vi "校准任务设置.vi"(10 "校准触发任务":refnum<user-event>, 11 "用户事件":refnum<user-event>) -> ()   [LabVIEW 2016, in "斯坦道CODMn新电路板.lvlib"]
uses:
  <vilib>/Utility/xml.llb/Write to XML File(string).vi
  <vilib>/Utility/xml.llb/Read From XML File(string).vi
panel:
  in  "导入":bool
  in  "保存":bool
  in  "校准任务存档":T1[](array[typedef])
  out "字符串":string
  out "校准运行状态":bool
  in  "校准任务":T1[](array[typedef])
  in  "停止":bool
  in  "设置":bool
  in  "执行":bool
  in  "删除":bool
  in  "清空":bool
  in  "任务列表":i32(listbox)
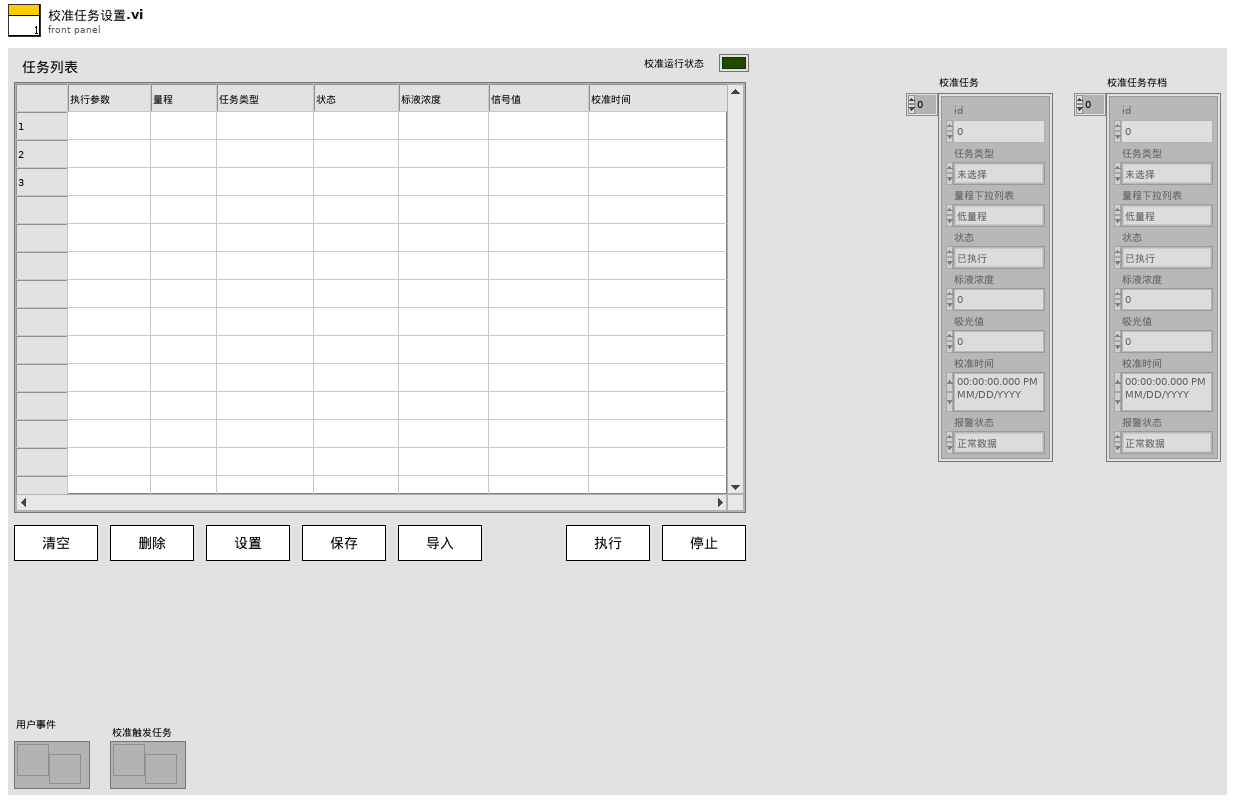
[diagram p1: front panel]
types:
  T1 = typedef "校准任务.ctl" = cluster{"id":u16, "任务类型":enum16{"未选择", "空白校准", "标样校准", "标样核查", "零点核查", "跨度核查"}, "量程下拉列表":enum16{"低量程", "高量程"}, "状态":enum16{"已执行", "待执行", "执行中", "停止"}, "标液浓度":dbl, "吸光值":dbl, "校准时间":timestamp, "报警状态":enum16{"正常数据", "报警数据"}}
  T2 = cluster{"校准类型":string, "校准数据":cluster{"时间":timestamp, "标液值":dbl, "检测值":dbl, "吸光值":dbl}}
  T3 = enum8{"Enabled", "Disabled", "Disabled and Grayed Out"}
  T4 = typedef "LVPoint32TypeDef.ctl" = cluster{"Horizontal":i32, "Vertical":i32}
  T5 = typedef "LVRowAndColumnTypeDef.ctl" = cluster{"Row":i32, "Column":i32}
  T6 = enum16{"未选择", "空白校准", "标样校准", "标样核查", "零点核查", "跨度核查"}
  T7 = cluster{"id":u16, "任务类型":enum16{"未选择", "空白校准", "标样校准", "标样核查", "零点核查", "跨度核查"}, "量程下拉列表":enum16{"低量程", "高量程"}, "状态":enum16{"已执行", "待执行", "执行中", "停止"}, "标液浓度":dbl, "吸光值":dbl, "校准时间":timestamp, "报警状态":enum16{"正常数据", "报警数据"}}
  T8 = enum32{"Bad", "Idle", "Run top level", "Running"}
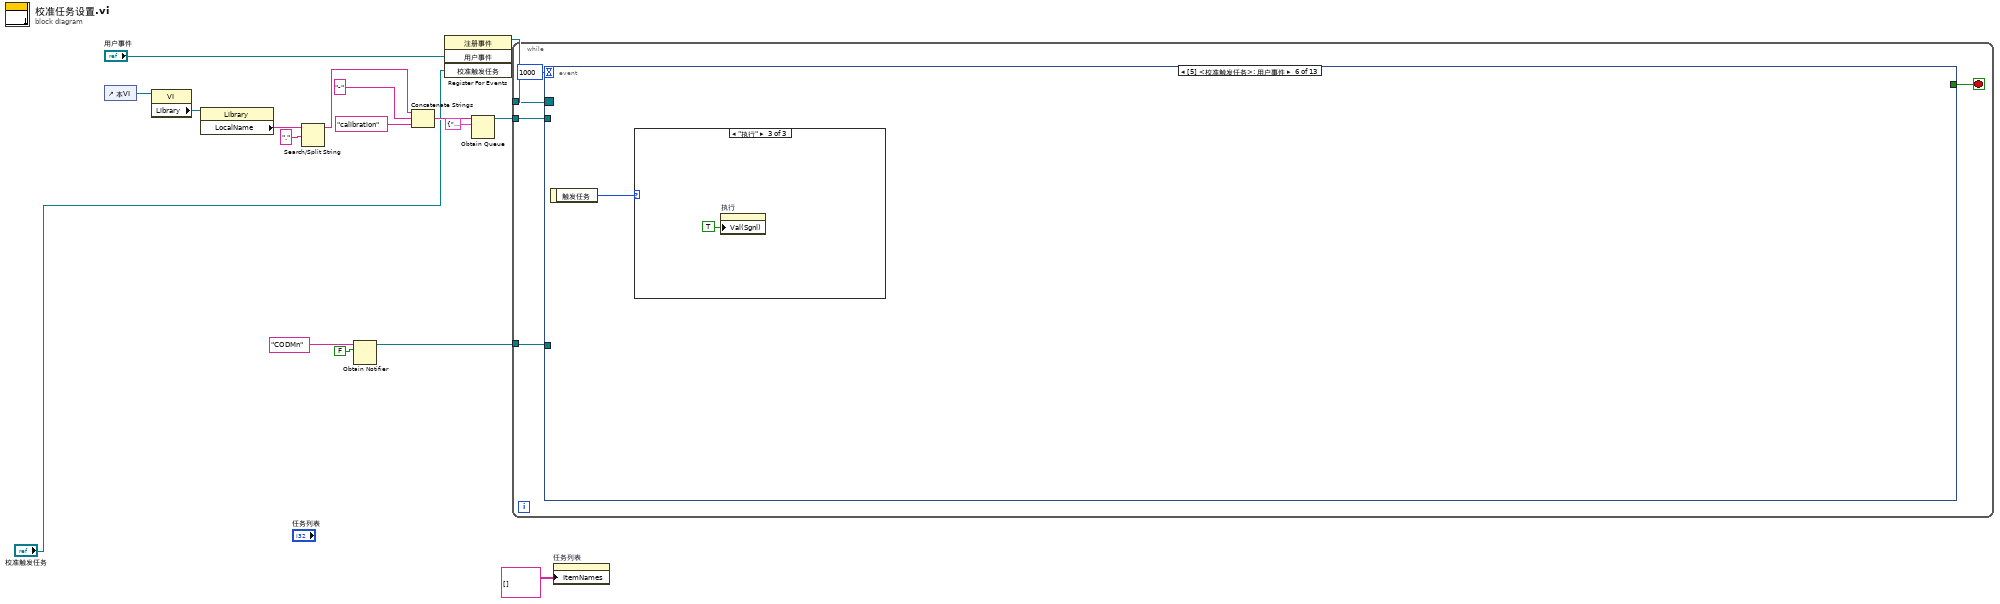
[diagram p0: block diagram]
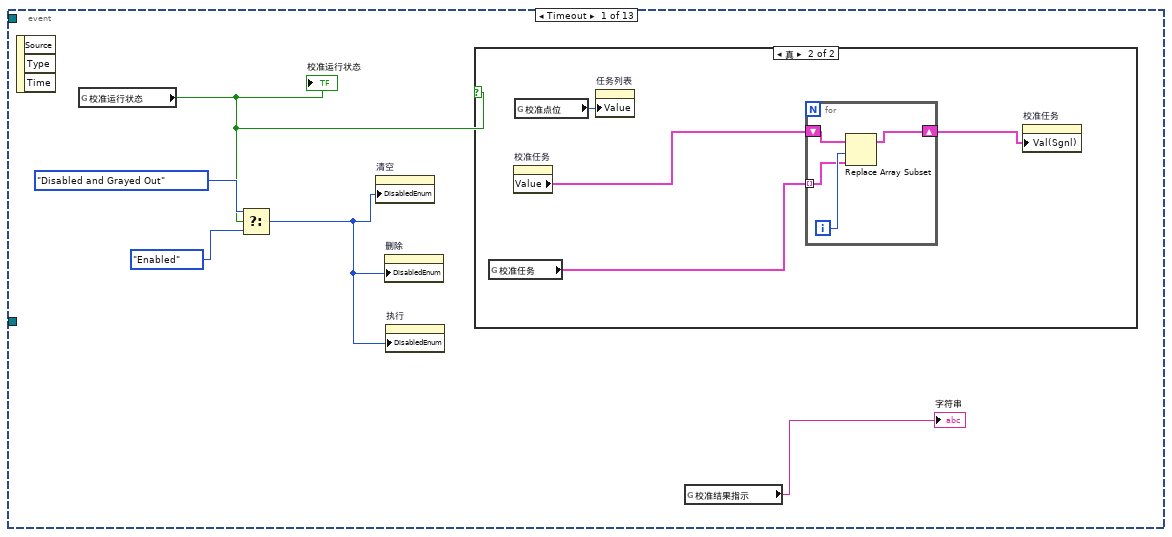
[diagram p2: hidden frame]
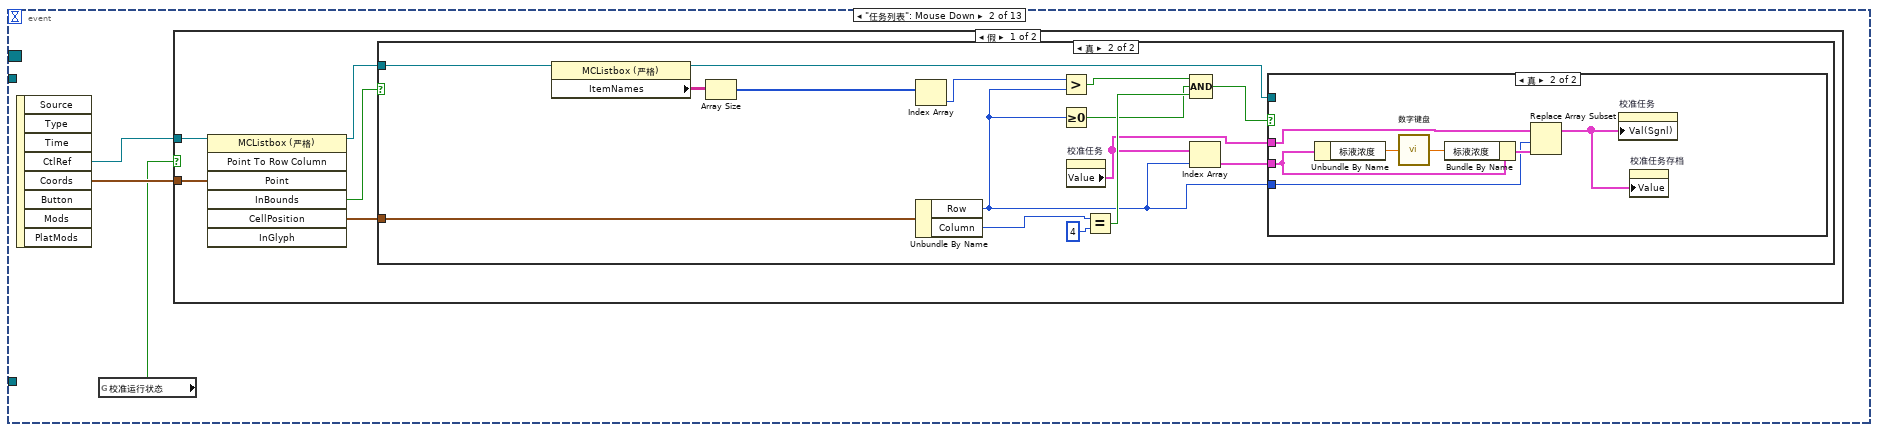
[diagram p4: hidden frame]
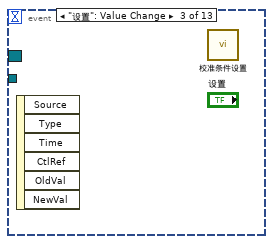
[diagram p8: hidden frame]
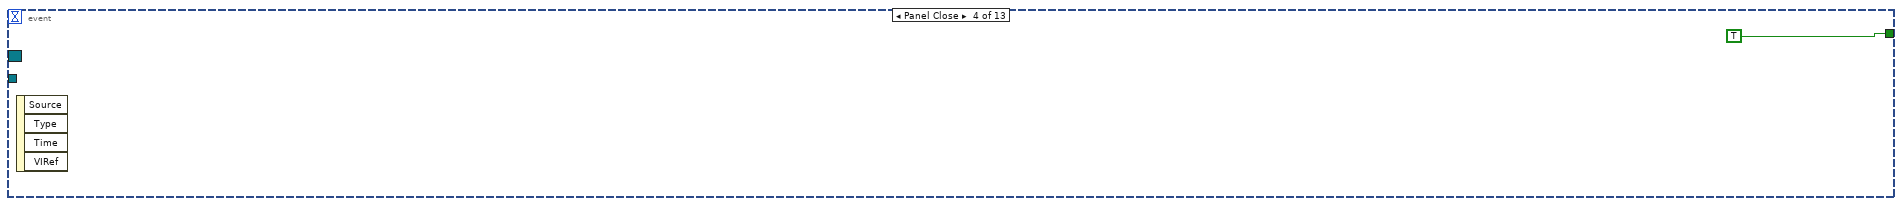
[diagram p9: hidden frame]
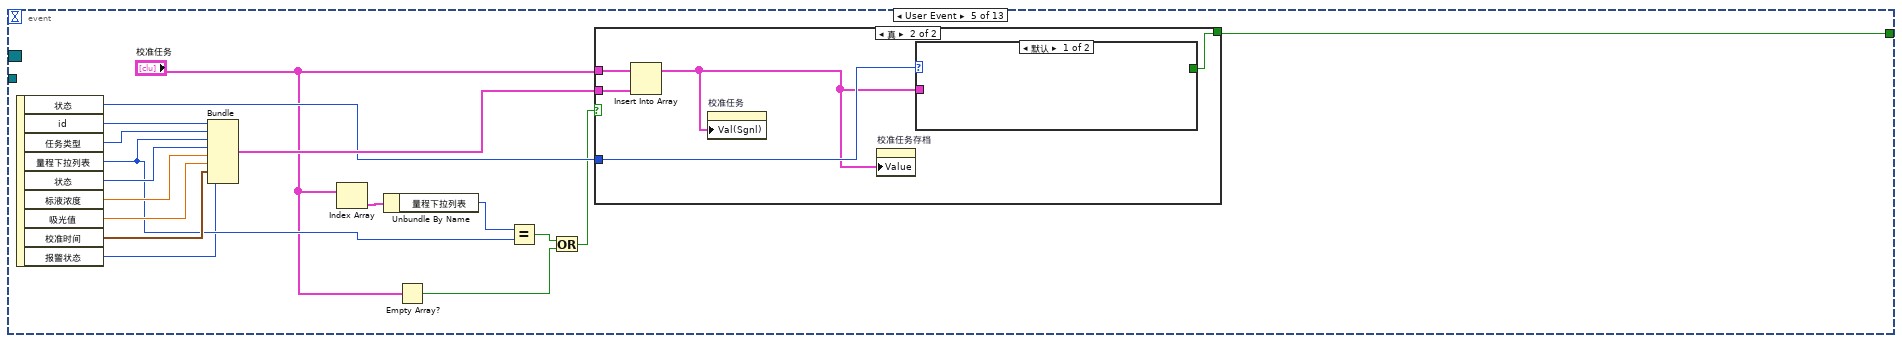
[diagram p10: hidden frame]
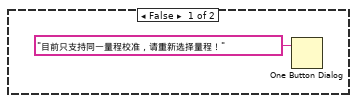
[diagram p11: hidden frame]
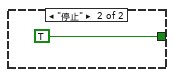
[diagram p12: hidden frame]
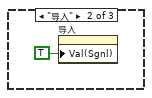
[diagram p14: hidden frame]
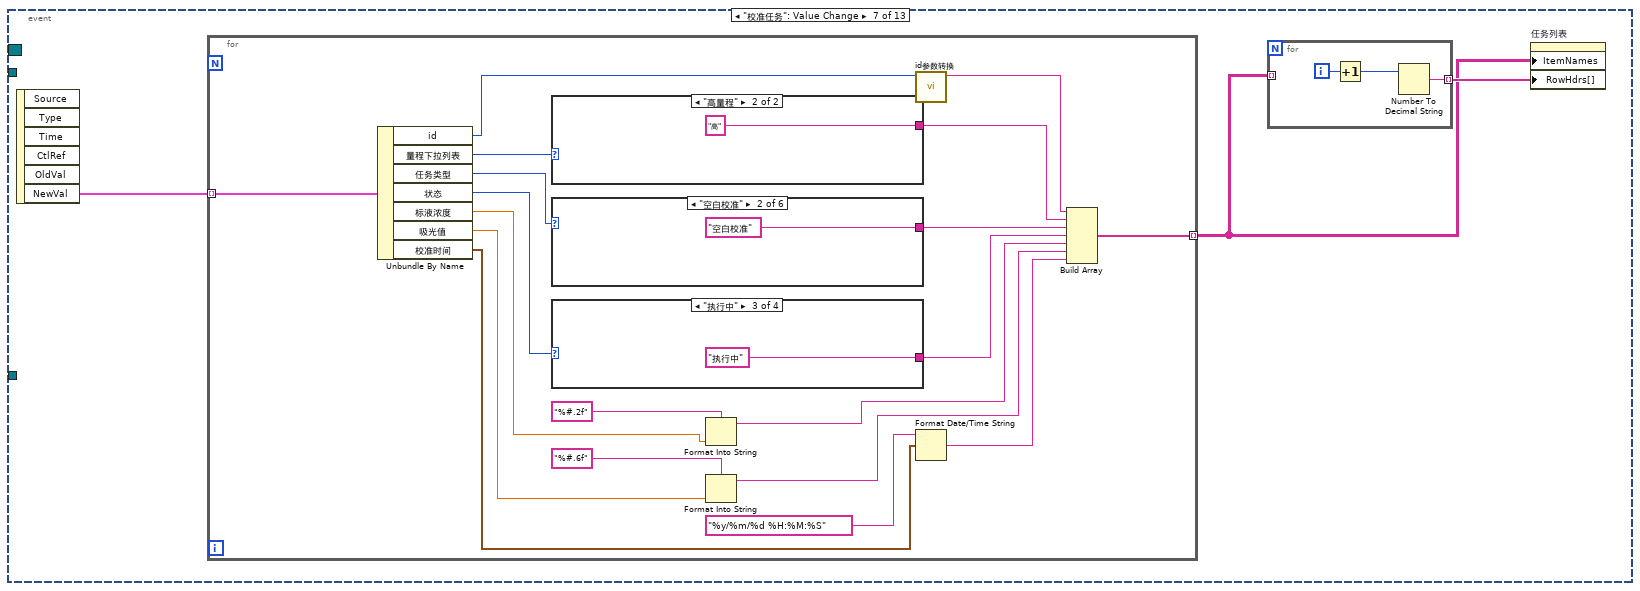
[diagram p15: hidden frame]
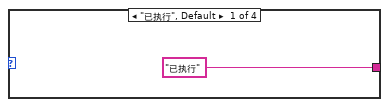
[diagram p16: hidden frame]
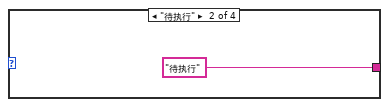
[diagram p17: hidden frame]
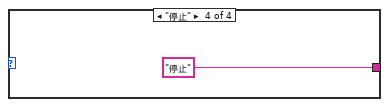
[diagram p18: hidden frame]
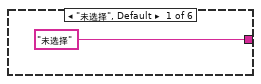
[diagram p19: hidden frame]
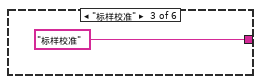
[diagram p20: hidden frame]
diagram:
  n1 = control-ref of="本VI"() -> (w16:refnum<vi>)
  n2 = property class="VI"(reference=w16) -> ("Library"=w17:refnum<vi>)  [unwired: 1 in, 2 out]
  n3 = property class="Library"(reference=w17) -> ("LocalName"=w15:string)  [unwired: 1 in, 2 out]
  n4 = Search/Split String(string=w15, search string/char (-)="." ("搜索字符串/字符(-)")) -> (substring before match=w13:string)  [unwired: 1 in, 2 out]
  n5 = Obtain Notifier(name (unnamed)="CODMn" ("字符串"), notification data type=FALSE) -> (notifier out=w4:refnum<notifier>)  [unwired: 2 in, 2 out]
  n6 = Concatenate Strings(w13, "-" ("字符串"), "calibration" ("名称或相对路径")) -> (w10:string)
  n7 = register-events("用户事件", "校准触发任务") -> (reference out=w7:refnum<event-registration>)  [unwired: 2 in, 1 out]
  n8 = Obtain Queue(name (unnamed)=w10, element data type=T2 {"校准类型"="", "校准数据"={"时间"=timestamp(0 s since 1904-01-01), "标液值"=0.0, "检测值"=0.0, "吸光值"=0.0}}) -> (queue out=w8:refnum<queue>)  [unwired: 3 in, 2 out]
  n9 = while {
    tunnel: w8 -> [w21]
    tunnel: w7 -> [w20]
    tunnel: w4 -> [w19]
    stop <- w22 stop-if-true
    n10 = event shown="[5] <校准触发任务>: 用户事件" {
      selector: w20 -> [_ _ _ _ _ _ _ _ _ _ _ _ _]
      dyn-events: _ -> [_ _ _ _ _ _ _ _ _ _ _ _ _]
      timeout: 1000 -> [_ _ _ _ _ _ _ _ _ _ _ _ _]
      tunnel: [_ _ _ TRUE w83 _ _ _ _ _ _ _ _] -> w22
      tunnel: w21 -> [_ _ _ _ _ _ _ _ _ _ _ _ _]
      tunnel: w19 -> [_ _ _ _ _ _ _ _ _ _ w153 _ _]
      event Timeout {
        n11 = event-data() -> ()  [unwired: 1 in, 3 out]
        n12 = global read "VARCODMn全局变量.vi" "校准运行状态"() -> (w24:bool)
        "校准运行状态" <- w24
        n13 = Select(t=T3."Disabled and Grayed Out" ("禁用"), s=w24, f=T3."Enabled" ("禁用")) -> (s? t:f=w26:T3)
        n14 = property on="清空" class="Bool"("DisabledEnum"=w26) -> ()  [unwired: 2 in, 2 out]
        n15 = property on="删除" class="Bool"("DisabledEnum"=w26) -> ()  [unwired: 2 in, 2 out]
        n16 = property on="执行" class="Bool (严格)"("DisabledEnum"=w26) -> ()  [unwired: 2 in, 2 out]
        n17 = case shown="真" w24 {
          frame False {
          }
          frame True {
            n18 = global read "VARCODMn全局变量.vi" "校准任务"() -> (w29:T1[])
            n19 = property on="校准任务" class="Arr (严格)"() -> ("Value"=w30:T1[])  [unwired: 2 in, 2 out]
            n20 = global read "VARCODMn全局变量.vi" "校准点位"() -> (w31:u16)
            n21 = property on="任务列表" class="MCListbox (严格)"("Value"=w31) -> ()  [unwired: 2 in, 2 out]
            n22 = for {
              tunnel: w29 -> [w33] mode=indexing
              shift-right: [w32] -> w28
              shift-left: w30 -> [w35]
              i -> [w34]
              n23 = Replace Array Subset(array=w35, new element=w33, index=w34) -> (w32:T1[])
            }
            n24 = property on="校准任务" class="Arr (严格)"("Val(Sgnl)"=w28) -> ()  [unwired: 2 in, 2 out]
          }
        }
        n25 = global read "VARCODMn全局变量.vi" "校准结果指示"() -> (→"字符串":string)
      }
      event "任务列表": Mouse Down {
        n26 = event-data() -> ("CtlRef"=w38:refnum<vi>, "Coords"=w37:T4)  [unwired: 1 in, 6 out]
        n27 = global read "VARCODMn全局变量.vi" "校准运行状态"() -> (w36:bool)
        n28 = case shown="假" w36 {
          tunnel: w38 -> [w43 _]
          tunnel: w37 -> [w39 _]
          frame False {
            n29 = invoke class="MCListbox (严格)" method="Point To Row Column"(reference=w43, "Point"=w39) -> (reference out=w40:refnum<vi>, "InBounds"=w42:bool, "CellPosition"=w41:T5)  [unwired: 5 in, 4 out]
            n30 = case shown="真" w42 {
              tunnel: w41 -> [_ w58]
              tunnel: w40 -> [_ w57]
              frame False {
              }
              frame True {
                n31 = property class="MCListbox (严格)"(reference=w57) -> (reference out=w56:refnum<vi>, "ItemNames"=w55:string[][])  [unwired: 1 in, 1 out]
                n32 = Array Size(array=w55) -> (size(s)=w54:i32[])
                n33 = Index Array(array=w54) -> (element=w53:i32)  [unwired: 1 in]
                n34 = Unbundle By Name(w58) -> ("Row"=w44:i32, "Column"=w52:i32)
                n35 = Greater?(x=w53, y=w44) -> (0:w48:bool)
                n36 = Greater Or Equal To 0?(x=w44) -> (x >= 0?=w47:bool)
                n37 = property on="校准任务" class="Arr (严格)"() -> ("Value"=w45:T1[])  [unwired: 2 in, 2 out]
                n38 = Equal?(x=w52, y=4) -> (x = y?=w50:bool)
                n39 = Compound Arithmetic op=AND ("复合运算")(w48, w47, w50) -> (w49:bool)
                n40 = Index Array(array=w45, index=w44) -> (element=w46:T1)
                n41 = case shown="真" w49 {
                  tunnel: w56 -> [_ _]
                  tunnel: w46 -> [_ w64]
                  tunnel: w45 -> [_ w62]
                  tunnel: w44 -> [_ w60]
                  frame False {
                  }
                  frame True {
                    n42 = Unbundle By Name(w64) -> ("标液浓度"=w65:dbl)
                    n43 = call "数字键盘.vi"("OldNumber"=w65) -> ("NewNumber"=w63:dbl)
                    n44 = Bundle By Name(cluster=w64, "标液浓度"=w63) -> (w61:T1)
                    n45 = Replace Array Subset(array=w62, new element=w61, index=w60) -> (w59:T1[])
                    n46 = property on="校准任务" class="Arr (严格)"("Val(Sgnl)"=w59) -> ()  [unwired: 2 in, 2 out]
                    n47 = property on="校准任务存档" class="Arr (严格)"("Value"=w59) -> ()  [unwired: 2 in, 2 out]
                  }
                }
              }
            }
          }
          frame True {
          }
        }
      }
      event "设置": Value Change {
        n48 = event-data() -> ()  [unwired: 1 in, 6 out]
        n49 = call "校准条件设置.vi"() -> ()  [unwired: 12 in]
      }
      event Panel Close {
        n50 = event-data() -> ()  [unwired: 1 in, 4 out]
      }
      event User Event {
        n51 = event-data() -> ("状态"=w75:enum16{"已执行", "待执行", "执行中", "停止"}, "id"=w82:u16, "任务类型"=w80:T6, "量程下拉列表"=w72:enum16{"低量程", "高量程"}, "状态"=w79:enum16{"已执行", "待执行", "执行中", "停止"}, "标液浓度"=w78:dbl, "吸光值"=w77:dbl, "校准时间"=w76:timestamp, "报警状态"=w67:enum16{"正常数据", "报警数据"})  [unwired: 1 in]
        n52 = Bundle("id"=w82, "任务类型"=w80, "量程下拉列表"=w72, "状态"=w79, "标液浓度"=w78, "吸光值"=w77, "校准时间"=w76, "报警状态"=w67) -> (w81:T7)  [unwired: 1 in]
        n53 = Index Array(array="校准任务") -> (element=w74:T1)  [unwired: 1 in]
        n54 = Unbundle By Name(w74) -> ("量程下拉列表"=w73:enum16{"低量程", "高量程"})
        n55 = Empty Array?(array="校准任务") -> (empty?=w68:bool)
        n56 = Equal?(x=w73, y=w72) -> (x = y?=w70:bool)
        n57 = Or(x=w70, y=w68) -> (x .or. y?=w69:bool)
        n58 = case shown="真" w69 {
          tunnel: [_ w89] -> w83
          tunnel: w81 -> [_ w88]
          tunnel: w75 -> [_ w87]
          tunnel: "校准任务" -> [_ w86]
          frame False {
            n59 = One Button Dialog(message="目前只支持同一量程校准，请重新选择量程！" ("消息")) -> ()  [unwired: 1 in, 1 out]
          }
          frame True {
            n60 = Insert Into Array(array=w86, new element=w88) -> (w85:T1[])  [unwired: 1 in]
            n61 = property on="校准任务" class="Arr (严格)"("Val(Sgnl)"=w85) -> ()  [unwired: 2 in, 2 out]
            n62 = property on="校准任务存档" class="Arr (严格)"("Value"=w85) -> ()  [unwired: 2 in, 2 out]
            n63 = case shown="默认" w87 {
              tunnel: [_ TRUE] -> w89
              tunnel: w85 -> [_ _]
              frame Default {
              }
              frame "停止" {
              }
            }
          }
        }
      }
      event User Event {
        n64 = event-data() -> ("触发任务"=w91:enum16{"Non", "导入", "执行"})  [unwired: 1 in]
        n65 = case shown="\"执行\"" w91 {
          frame "Non", Default {
          }
          frame "导入" {
            n66 = property on="导入" class="Bool (严格)"("Val(Sgnl)"=TRUE ("值(信号)")) -> ()  [unwired: 2 in, 2 out]
          }
          frame "执行" {
            n67 = property on="执行" class="Bool (严格)"("Val(Sgnl)"=TRUE ("值(信号)")) -> ()  [unwired: 2 in, 2 out]
          }
        }
      }
      event "校准任务": Value Change {
        n68 = event-data() -> ("NewVal"=w94:T1[])  [unwired: 1 in, 5 out]
        n69 = for {
          tunnel: w94 -> [w115] mode=indexing
          tunnel: [w97] -> w95 mode=indexing
          n70 = Unbundle By Name(w115) -> ("id"=w114:u16, "量程下拉列表"=w113:enum16{"低量程", "高量程"}, "任务类型"=w112:T6, "状态"=w111:enum16{"已执行", "待执行", "执行中", "停止"}, "标液浓度"=w109:dbl, "吸光值"=w107:dbl, "校准时间"=w105:timestamp)
          n71 = case shown="\"高量程\"" w113 {
            tunnel: ["低" "高"] -> w103
            frame "低量程", Default {
            }
            frame "高量程" {
            }
          }
          n72 = case shown="\"空白校准\"" w112 {
            tunnel: ["未选择" "空白校准" "标样校准" "标样核查" "零点核查" "跨度核查"] -> w102
            frame "未选择", Default {
            }
            frame "空白校准" {
            }
            frame "标样校准" {
            }
            frame "标样核查" {
            }
            frame "零点核查" {
            }
            frame "跨度核查" {
            }
          }
          n73 = case shown="\"执行中\"" w111 {
            tunnel: ["已执行" "待执行" "执行中" "停止"] -> w101
            frame "已执行", Default {
            }
            frame "待执行" {
            }
            frame "执行中" {
            }
            frame "停止" {
            }
          }
          n74 = Format Into String(format string="%#.2f" ("格式字符串"), w109) -> (resulting string=w100:string)  [unwired: 2 in, 1 out]
          n75 = Format Into String(format string="%#.6f" ("格式字符串"), w107) -> (resulting string=w99:string)  [unwired: 2 in, 1 out]
          n76 = call "id参数转换.vi"("id"=w114) -> ("table输出"=w104:string)  [unwired: 10 in]
          n77 = Format Date/Time String(time format string (%c)="%y/%m/%d %H:%M:%S" ("时间格式字符串(%c)"), seconds (now)=w105) -> (date/time string=w98:string)  [unwired: 1 in]
          n78 = Build Array(w104, w103, w102, w101, w100, w99, w98) -> (w97:string[])
        }
        n79 = for {
          tunnel: [w128] -> w96 mode=indexing
          tunnel: w95 -> [_] mode=indexing
          i -> [w130]
          n80 = Increment(x=w130) -> (x+1=w129:i32)
          n81 = Number To Decimal String(number=w129) -> (decimal integer string=w128:string)  [unwired: 1 in]
        }
        n82 = property on="任务列表" class="MCListbox (严格)"("ItemNames"=w95, "RowHdrs[]"=w96) -> ()  [unwired: 2 in, 2 out]
      }
      event "清空": Value Change {
        n83 = event-data() -> ()  [unwired: 1 in, 6 out]
        n84 = property on="校准任务" class="Arr (严格)"("Val(Sgnl)"=T1[] [] ("数组")) -> ()  [unwired: 2 in, 2 out]
      }
      event "删除": Value Change {
        n85 = event-data() -> ()  [unwired: 1 in, 6 out]
        n86 = property on="校准任务" class="Arr (严格)"() -> ("Value"=w134:T1[])  [unwired: 2 in, 2 out]
        n87 = property on="任务列表" class="MCListbox (严格)"() -> ("Value"=w132:i32)  [unwired: 2 in, 2 out]
        n88 = Delete From Array(array=w134, index=w132) -> (array with subset deleted=w133:T1[])  [unwired: 1 in, 1 out]
        n89 = property on="校准任务" class="Arr (严格)"("Val(Sgnl)"=w133) -> ()  [unwired: 2 in, 2 out]
      }
      event "执行": Value Change {
        n90 = event-data() -> ()  [unwired: 1 in, 6 out]
        n91 = local write "执行"(FALSE ("执行")) -> ()
        n92 = global read "VARCODMn全局变量.vi" "校准精度"() -> (w136:dbl)
        n93 = vi-ref "斯坦道CODMn新电路板.lvlib:校准任务流程.vi"() -> (w138:refnum<vi>)
        n94 = global read "VARCODMn全局变量.vi" "校准模型"() -> (w137:enum32{"线性", "多项式", "折线"})
        n95 = property class="VI"(reference=w138) -> (reference out=w141:refnum<vi>, "Name"=w139:string, "Exec.State"=w140:T8)  [unwired: 1 in, 1 out]
        n96 = case shown="\"Idle\"" w140 {
          tunnel: w139 -> [_ w151]
          tunnel: w141 -> [_ _]
          tunnel: w137 -> [_ w144]
          tunnel: w136 -> [_ w143]
          frame "Bad", Default {
          }
          frame "Idle" {
            n97 = Open VI Reference(type specifier VI Refnum (for type only)=refnum<vi> refnum, vi path=w151, options=128 ("选项")) -> (vi reference=w149:refnum<vi>, error out=w147:errorcluster)  [unwired: 3 in]
            n98 = call-by-ref "开始异步调用"(reference=w149, error in=w147, "校准任务"="校准任务存档", "精度"=w143, "模型"=w144) -> (reference out=w148:refnum<vi>, error out=w146:errorcluster)  [unwired: 9 in]
            n99 = Close Reference(reference=w148, error in (no error)=w146) -> ()  [unwired: 1 out]
          }
        }
      }
      event "停止": Value Change {
        n100 = event-data() -> ()  [unwired: 1 in, 6 out]
        n101 = Send Notification(notification=TRUE ("通知"), notifier=w153) -> ()  [unwired: 1 in, 2 out]
      }
      event "保存": Value Change {
        n102 = event-data() -> ()  [unwired: 1 in, 6 out]
        n103 = local write "保存"(FALSE ("保存")) -> ()
        n104 = property on="校准任务" class="Arr (严格)"() -> ("Value"=w155:T1[])  [unwired: 2 in, 2 out]
        n105 = for {
          tunnel: w155 -> [w170] mode=indexing
          tunnel: [w169] -> w158 mode=indexing
          n106 = in-place {
            n107 = in-place-cluster #1(w170) -> ()  [unwired: 1 out]
            n108 = in-place-cluster #1("状态"=enum16{"已执行", "待执行", "执行中", "停止"}."待执行") -> (w169:T1)
          }
        }
        n109 = control-ref of="本VI"() -> (w164:refnum<vi>)
        n110 = property class="VI"(reference=w164) -> ("Library"=w165:refnum<vi>)  [unwired: 1 in, 2 out]
        n111 = property class="Library"(reference=w165) -> ("LocalName"=w162:string)  [unwired: 1 in, 2 out]
        n112 = call <vilib>:"Application Directory.vi"() -> ("Application Directory"=w168:path)
        n113 = Search/Split String(string=w162, search string/char (-)="." ("搜索字符串/字符(-)")) -> (substring before match=w161:string)  [unwired: 1 in, 2 out]
        n114 = Build Path(base path=w168, name or relative path="config" ("名称或相对路径")) -> (appended path=w166:path)
        n115 = Concatenate Strings(w161, "CalTask.xml" ("字符串")) -> (w160:string)
        n116 = Build Path(base path=w166, name or relative path=w160) -> (appended path=w156:path)
        n117 = Flatten To XML(anything=w158) -> (xml string=w157:string)
        n118 = call-poly <vilib>:"Write to XML File.vi"("XML Input"=w157, "XML File Path"=w156) -> ()  [unwired: 7 in, 3 out]
      }
      event "导入": Value Change {
        n119 = event-data() -> ()  [unwired: 1 in, 6 out]
        n120 = local write "导入"(FALSE ("导入")) -> ()
        n121 = control-ref of="本VI"() -> (w182:refnum<vi>)
        n122 = property class="VI"(reference=w182) -> ("Library"=w183:refnum<vi>)  [unwired: 1 in, 2 out]
        n123 = property class="Library"(reference=w183) -> ("LocalName"=w180:string)  [unwired: 1 in, 2 out]
        n124 = call <vilib>:"Application Directory.vi"() -> ("Application Directory"=w186:path)
        n125 = Search/Split String(string=w180, search string/char (-)="." ("搜索字符串/字符(-)")) -> (substring before match=w179:string)  [unwired: 1 in, 2 out]
        n126 = Build Path(base path=w186, name or relative path="config" ("名称或相对路径")) -> (appended path=w184:path)
        n127 = Concatenate Strings(w179, "CalTask.xml" ("字符串")) -> (w178:string)
        n128 = Build Path(base path=w184, name or relative path=w178) -> (appended path=w176:path)
        n129 = local read "校准任务"() -> (w174:T1[])
        n130 = call-poly <vilib>:"Read From XML File.vi"("XML File Path"=w176) -> ("XML Elements"=w175:string)  [unwired: 8 in, 2 out]
        n131 = Unflatten From XML(xml string=w175, type=w174) -> (value=w172:T1[])  [unwired: 1 in, 1 out]
        n132 = property on="校准任务存档" class="Arr (严格)"("Value"=w172) -> ()  [unwired: 2 in, 2 out]
        n133 = property on="校准任务" class="Arr (严格)"("Val(Sgnl)"=w172) -> ()  [unwired: 2 in, 2 out]
      }
    }
  }
  n134 = property on="任务列表" class="MCListbox (严格)"("ItemNames"=string[][] [] ("项名")) -> ()  [unwired: 2 in, 2 out]
